vi "Initialize and Sort Key Values.vi"() -> (8 "refnum":T1, 11 "Preferences":string[][](array[string]))   [LabVIEW 2015]
uses:
  <vilib>/Utility/config.llb/Config Data RefNum.ctl
  <vilib>/Rock Robotics/Network Tables/NT Read String.vi
  <vilib>/Utility/config.llb/Read Key (String).vi
  <vilib>/Utility/config.llb/NI_LVConfig.lvlib
panel:
  out "error out":errorcluster
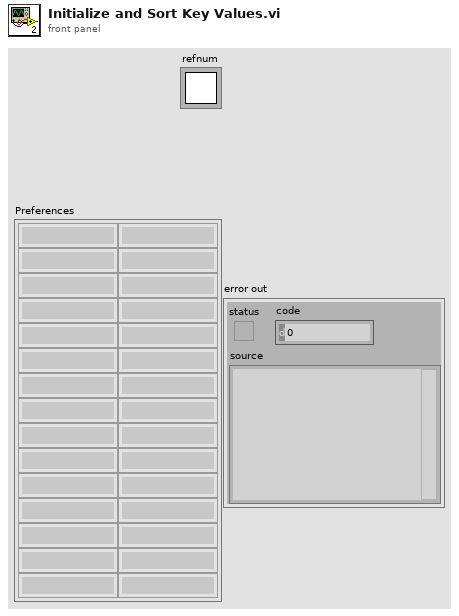
[diagram p1: front panel]
types:
  T1 = typedef "NI_LVConfig.lvlib/Config Data RefNum.ctl" = refnum<k1>
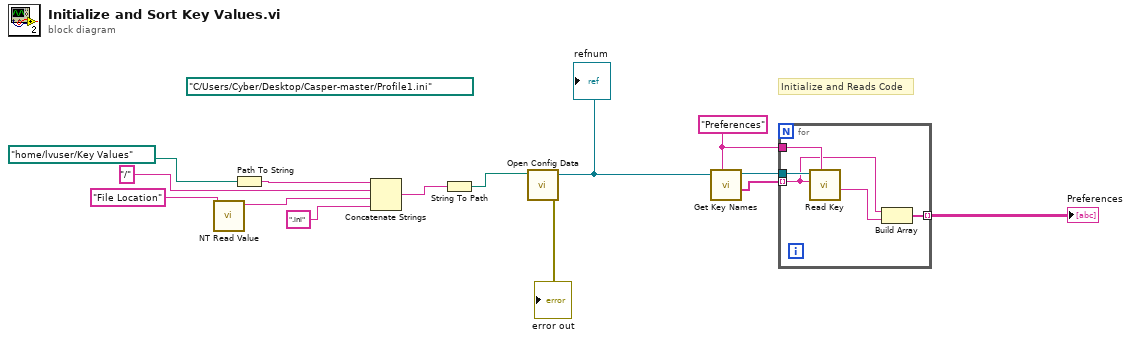
[diagram p0: block diagram]
diagram:
  (unwired) path "C:/Users/Cyber/Desktop/Casper-master/Profile1.ini" ("path")
  w13 = "Preferences" ("section")
  # "Initialize and Reads Code"
  n1 = call-poly <vilib>:"NT Read Value.vi"("Name"="File Location") -> ("String"=w2:string)  [unwired: 9 in, 1 out]
  n2 = Path To String(path=path "/home/lvuser/Key Values" ("configuration file path")) -> (string=w9:string)
  n3 = Concatenate Strings(w9, "/" ("string"), w2, ".ini" ("string")) -> (w8:string)
  n4 = String To Path(string=w8) -> (path=w1:path)
  n5 = call <vilib>:"Open Config Data.vi"("configuration file path"=w1) -> ("error out"=→"error out":errorcluster, "refnum"=w11:T1)  [unwired: 8 in, 1 out]
  "refnum" <- w11
  n6 = call <vilib>:"Get Key Names.vi"("section"=w13, "refnum"=w11) -> ("key names"=w14:string[], "refnum out"=w12:T1)  [unwired: 6 in, 2 out]
  n7 = for {
    tunnel: w14 -> [w17] mode=indexing
    tunnel: w12 -> [w19]
    tunnel: w13 -> [w18]
    tunnel: [w15] -> w10 mode=indexing
    n8 = call-poly <vilib>:"Read Key.vi"("section"=w18, "key"=w17, "refnum"=w19) -> ("value"=w16:string)  [unwired: 5 in, 3 out]
    n9 = Build Array(w17, w16) -> (w15:string[])
  }
  "Preferences" <- w10
